vi "20220815-335-write temppoint.vi"() -> ()   [LabVIEW 2019]
doc: "This example VI demonstrates the proper use of the Configure Curve Header and Configure Curve Point VIs. It allows the user to write a curve header, a curve point, of both."
panel:
  out "当前已经写入（点数）":i32
  in  "曲线序号":string="59"
  in  "VISA resource name":refnum<visa-resource-name>
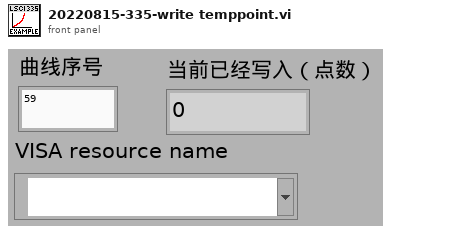
[diagram p1: front panel]
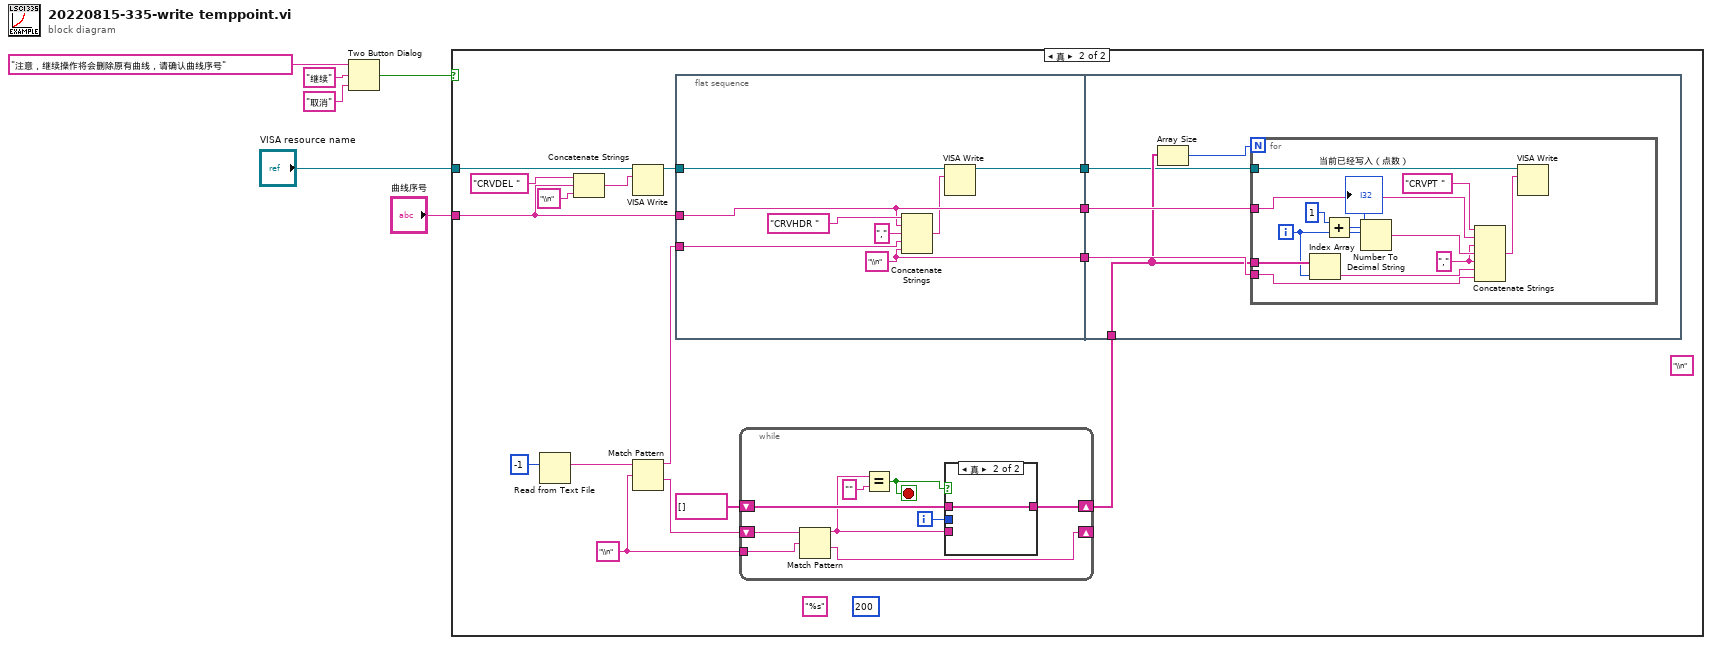
[diagram p0: block diagram]
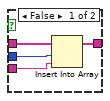
[diagram p3: hidden frame]
diagram:
  n1 = Two Button Dialog(message="注意，继续操作将会删除原有曲线，请确认曲线序号", 1:"取消" ("F button name (\"Cancel\")"), 2:"继续" ("T button name (\"OK\")")) -> (T button?=w6:bool)
  n2 = case shown="真" w6 {
    tunnel: "曲线序号" -> [_ w15]
    tunnel: "VISA resource name" -> [_ w10]
    frame False {
    }
    frame True {
      (unwired) 200
      (unwired) "%s" ("format string")
      (unwired) "\\n" ("delimiter (Tab)")
      w13 = "\\n" ("regular expression")
      n3 = Read from Text File(count=-1) -> (text=w21:string)  [unwired: 3 in, 3 out]
      n4 = Concatenate Strings("CRVDEL " ("string"), w15, "\\n" ("string")) -> (w8:string)
      n5 = VISA Write(VISA resource name=w10, write buffer=w8) -> (VISA resource name out=w9:refnum<visa-resource-name>)  [unwired: 1 in, 2 out]
      n6 = Match Pattern(string=w21, regular expression=w13) -> (before substring=w20:string, after substring=w14:string)  [unwired: 1 in, 2 out]
      n7 = flat-sequence {
        tunnel: w20 -> [w42]
        tunnel: [w40] -> w19
        tunnel: [w41] -> w18
        tunnel: w15 -> [w40]
        tunnel: w9 -> [w39]
        tunnel: [w37] -> w7
        tunnel: w19 -> [w49]
        tunnel: w18 -> [w48]
        tunnel: w11 -> [w47]
        tunnel: w7 -> [w45]
        frame #0 {
          w41 = "\\n" ("string")
          n8 = Concatenate Strings("CRVHDR " ("write buffer"), w40, "," ("string"), w42, w41) -> (w38:string)
          n9 = VISA Write(VISA resource name=w39, write buffer=w38) -> (VISA resource name out=w37:refnum<visa-resource-name>)  [unwired: 1 in, 2 out]
        }
        frame #1 {
          n10 = Array Size(array=w47) -> (size(s)=w46:i32)
          n11 = for {
            N: w46 -> [_]
            tunnel: w47 -> [w61]
            tunnel: w49 -> [w56]
            tunnel: w48 -> [w52]
            tunnel: w45 -> [w51]
            i -> [w54]
            w55 = "," ("string")
            n12 = Index Array(array=w61, index=w54) -> (element=w53:string)
            n13 = Add(x=1, y=w54) -> (x+y=w58:i32)
            n14 = Number To Decimal String(number=w58) -> (decimal integer string=w57:string)  [unwired: 1 in]
            n15 = Concatenate Strings("CRVPT " ("string"), w56, w55, w57, w55, w53, w52) -> (w50:string)
            n16 = VISA Write(VISA resource name=w51, write buffer=w50) -> ()  [unwired: 1 in, 3 out]
            "当前已经写入（点数）" <- w54
          }
        }
      }
      n17 = while {
        shift-right: [w29] -> _
        shift-left: w14 -> [w31]
        tunnel: w13 -> [w30]
        shift-right: [w26] -> w11
        shift-left: string[] [] ("after substring 2") -> [w28]
        i -> [w27]
        stop <- w23 stop-if-true
        n18 = Match Pattern(string=w31, regular expression=w30) -> (before substring=w25:string, after substring=w29:string)  [unwired: 1 in, 2 out]
        n19 = Equal?(x=w25, y="") -> (x = y?=w23:bool)
        n20 = case shown="真" w23 {
          tunnel: w28 -> [w35 w36]
          tunnel: w27 -> [w34 _]
          tunnel: [w33 w36] -> w26
          tunnel: w25 -> [w32 _]
          frame False {
            n21 = Insert Into Array(array=w35, index=w34, new element=w32) -> (w33:string[])
          }
          frame True {
          }
        }
      }
    }
  }
